vi "Set Geocode.vi"(0 "GMaps API in":refnum<class "GMaps API.lvclass">, 1 "Marker":T1={"Marker Color"="", "Marker Size "="", "Marker Label"="", "Marker State"="", "Marker City"=" ", "Marker Street"=""}, 5 "error in (no error)":errorcluster) -> (14 "GMaps API out":refnum<class "GMaps API.lvclass">, 19 "error out":errorcluster)   [LabVIEW 2016, in "GMaps API.lvclass"]
doc: "Sets converted addresses (like a street address) into geographic coordinates."
uses:
  GMaps API.lvclass
  Controls/Marker.ctl
  GMaps API.lvclass/GMaps API.ctl
  <vilib>/regexp/Match Regular Expression.xnode
  <vilib>/httpClient/LabVIEWHTTPClient.lvlib
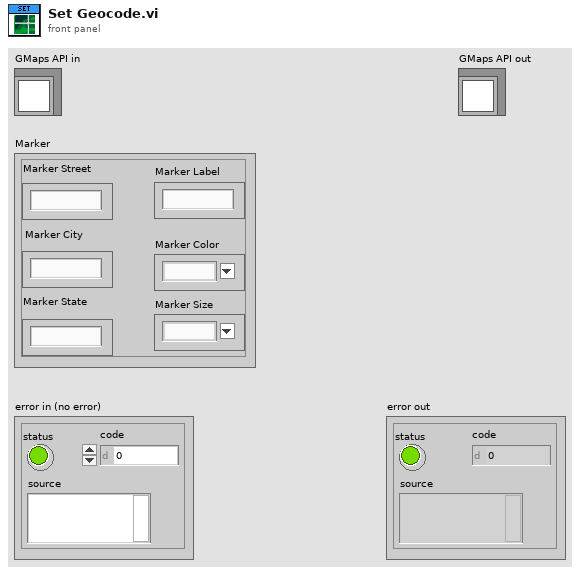
[diagram p1: front panel]
types:
  T1 = typedef "GMaps API.lvclass/Marker.ctl" = cluster{"Marker Color":string, "Marker Size ":string, "Marker Label":string, "Marker State":string, "Marker City":string, "Marker Street":string}
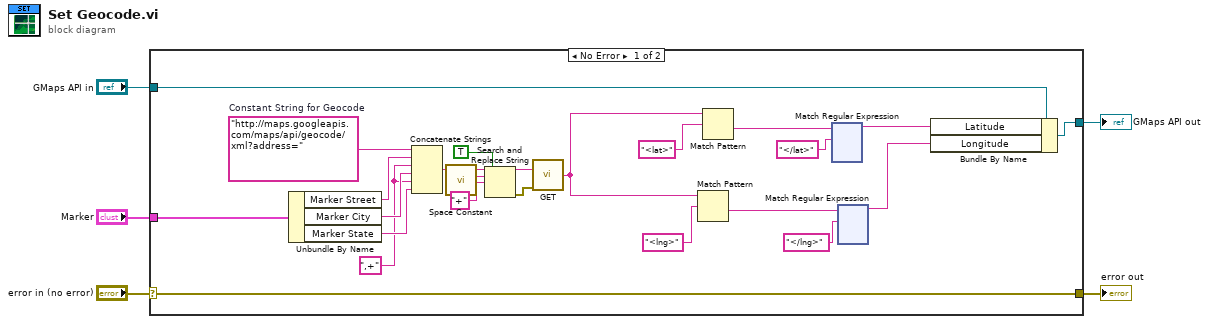
[diagram p0: block diagram]
diagram:
  n1 = case shown="No Error" "error in (no error)" {
    selector: "error in (no error)" -> [w29 w259]
    tunnel: [w29 w259] -> w4
    tunnel: [w6 w258] -> w2
    tunnel: "GMaps API in" -> [w9 w258]
    tunnel: "Marker" -> [w28 _]
    frame No Error {
      w10 = ",+" ("string")
      w25 = "http://maps.googleapis.com/maps/api/geocode/xml?address="  # Constant String for Geocode
      n2 = Unbundle By Name(w28) -> ("Marker Street"=w13:string, "Marker City"=w12:string, "Marker State"=w11:string)
      n3 = Concatenate Strings(w25, w13, w10, w12, w10, w11) -> (w24:string)
      n4 = call <vilib>:"Space Constant.vi"() -> ("String"=w23:string)
      n5 = Search and Replace String(replace all?=TRUE ("replace all? (F)"), input string=w24, search string=w23, replace string="+" ("replace string (\"\")")) -> (result string=w20:string, error out=w21:errorcluster)  [unwired: 4 in, 2 out]
      n6 = call <vilib>:"GET.vi"("url"=w20, "error in (no error)"=w21) -> ("body"=w16:string)  [unwired: 10 in, 3 out]
      n7 = Match Pattern(string=w16, regular expression="<lng>" ("Directly Before Latitude info")) -> (after substring=w14:string)  [unwired: 4 out]
      n8 = Match Pattern(string=w16, regular expression="<lat>") -> (after substring=w15:string)  [unwired: 4 out]
      n9 = xnode "Match Regular Expression"("input string"=w15, "regular expression"="</lat>") -> ("before match"=w8:string)  [unwired: 4 in, 4 out]
      n10 = xnode "Match Regular Expression"("input string"=w14, "regular expression"="</lng>" ("Directly After Latitude info")) -> ("before match"=w7:string)  [unwired: 4 in, 4 out]
      n11 = Bundle By Name(cluster=w9, "Latitude"=w8, "Longitude"=w7) -> (w6:refnum<class "GMaps API.lvclass">)
    }
    frame Error {
    }
  }
  "error out" <- w4
  "GMaps API out" <- w2
